vi "niRFUtil MASMT Flat Top Window (DBL).vi"(8 "error in (no error)":errorcluster, 11 "X":dbl[](array[numeric])) -> (0 "error out":errorcluster, 3 "Windowed X":dbl[](array[numeric]))   [LabVIEW 2015, in "niRFUtil.lvlib"]
doc: "Applies a flat top window to the input sequence <B>X</B>."
uses:
  niRFUtil.lvlib
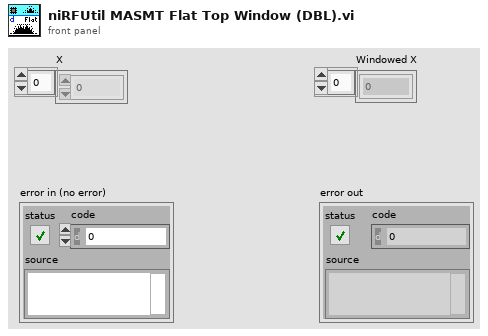
[diagram p1: front panel]
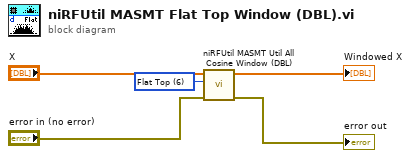
[diagram p0: block diagram]
diagram:
  w3 = 6 items=["None"=0, "Hanning"=1, "Hamming"=2, "Blackman-Harris"=3, "Exact Blackman"=4, "Blackman"=5, "Flat Top"=6, "4 Term B-Harris"=7, "7 Term B-Harris"=8, "Low Sidelobe"=9, "Blackman Nuttall"=11] ("cosine window")
  n1 = call "niRFUtil MASMT Util All Cosine Window (DBL).vi"("error in (no error)"="error in (no error)", "cosine window"=w3, "X"="X") -> ("error out"=→"error out":errorcluster, "Windowed X"=→"Windowed X":dbl[])  [unwired: 7 in]
